vi "niRFUtil RFHS Convert Voltage to dBm (complex array).vi"(0 "Complex Array (V)":T2 format="%.2f") -> (4 "Real Array (dBm)":T1 min=0 max=127 format="%.2f")   [LabVIEW 2015, in "niRFUtil.lvlib"]
uses:
  niRFUtil.lvlib
  Includes/niRFUtil INC Complex Array.ctl
  Includes/niRFUtil INC Real Array.ctl
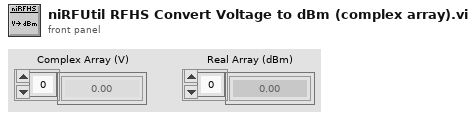
[diagram p1: front panel]
types:
  T1 = typedef "niRFUtil.lvlib/niRFUtil INC Real Array.ctl" = sgl[]
  T2 = typedef "niRFUtil.lvlib/niRFUtil INC Complex Array.ctl" = csg[]
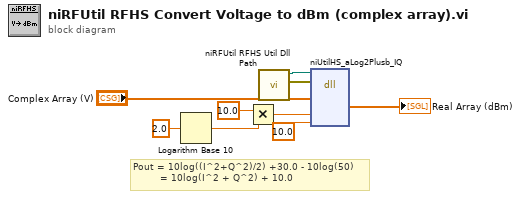
[diagram p0: block diagram]
diagram:
  # "Pout = 10log((I^2+Q^2)/2) +30.0 - 10log(50)\n         = 10log(I^2 + Q^2) + 10.0"
  n1 = Logarithm Base 10(1:sgl 2.0 ("x")) -> (0:w5:sgl)
  n2 = Multiply(x=sgl 10.0, y=w5) -> (x*y=w4:sgl)
  n3 = call "niRFUtil RFHS Util Dll Path.vi"() -> ("error out"=w1:errorcluster, "Path"=w2:path)  [unwired: 7 in, 3 out]
  n4 = dll-call lib="niRFHS_avx.*" fn="niUtilHS_aLog2Plusb_IQ" label="a*log2(x)+b"(path in=w2, error in=w1, "iBuf"="Complex Array (V)", "a"=w4, "b"=sgl 10.0) -> ("oBuf"=→"Real Array (dBm)":sgl[])  [unwired: 6 in, 2 out]
